vi "classify error.vi"(8 "error to classify":errorcluster, 10 "attempt recovery?":bool, 11 "TDMS datalogger runtime in":refnum<class "TDMS datalogger runtime.lvclass">) -> (0 "classified error":errorcluster, 2 "error classification":T1, 3 "TDMS datalogger runtime out":refnum<class "TDMS datalogger runtime.lvclass">)   [LabVIEW 2013, in "TDMS datalogger runtime.lvclass"]
doc: "Allows a module to classify an error generated at any point during execution. This <b>error classification</b> can then be used by calling code to determine if execution can continue. In addition, this function can be used to allow a component to clear an error, convert an error to a warning, or attempt to recover from an error. Recovery may be attempted only if <b>attempt recovery?</b> is true."
uses:
  TDMS datalogger runtime.lvclass
  <vilib>/NI/Tag Bus Module Framework/runtime/error classification.ctl
  <vilib>/NI/Tag Bus Module Framework/runtime/TBM module execution interface.lvclass
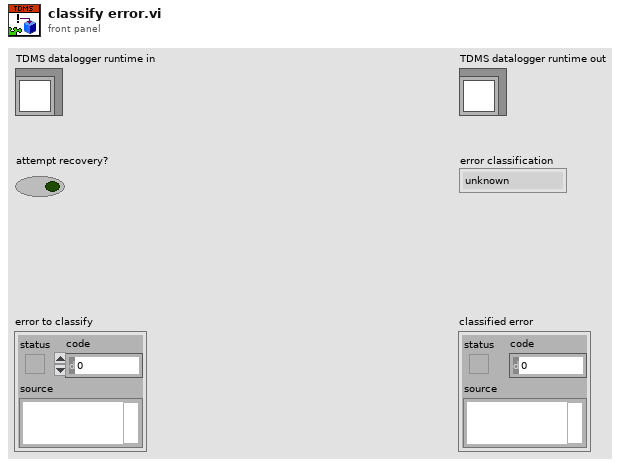
[diagram p1: front panel]
types:
  T1 = typedef "TBM module execution interface.lvclass/error classification.ctl" = enum16{"unknown", "none", "trivial", "recoverable", "critical"}
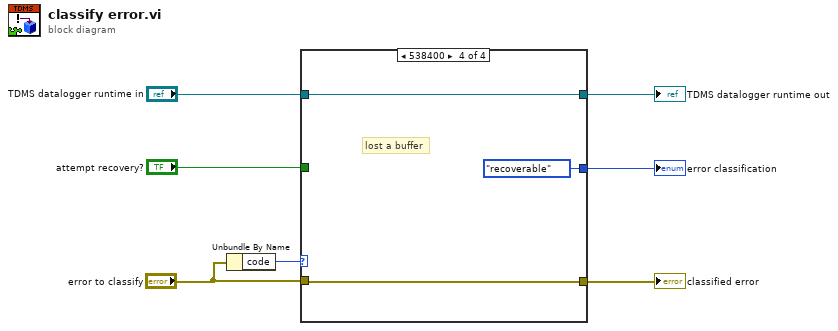
[diagram p0: block diagram]
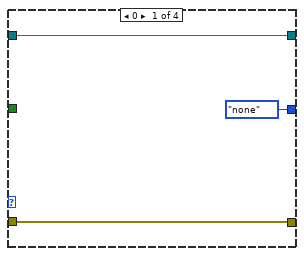
[diagram p2: hidden frame]
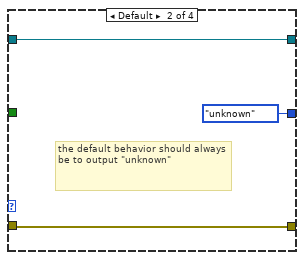
[diagram p3: hidden frame]
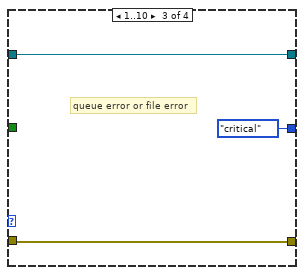
[diagram p4: hidden frame]
diagram:
  n1 = Unbundle By Name("error to classify") -> ("code"=w1:i32)
  n2 = case shown="538400" w1 {
    tunnel: "error to classify" -> [w9 w11 w14 w17]
    tunnel: [w9 w11 w14 w17] -> w3
    tunnel: [error_classification."none" ("error classification") error_classification."unknown" ("error classification") error_classification."critical" ("error classification") error_classification."recoverable" ("error classification")] -> w2
    tunnel: "TDMS datalogger runtime in" -> [w10 w12 w15 w18]
    tunnel: [w10 w12 w15 w18] -> w5
    tunnel: "attempt recovery?" -> [_ _ _ _]
    frame 0 {
    }
    frame Default {
      # "the default behavior should always be to output \"unknown\""
    }
    frame 1..10 {
      # "queue error or file error"
    }
    frame 538400 {
      # "lost a buffer"
    }
  }
  "TDMS datalogger runtime out" <- w5
  "error classification" <- w2
  "classified error" <- w3
